vi "Remove Extra Blines.vi"(6 "Data In":u16[][](array[numeric]), 8 "#Aline":i32=400, 9 "Start index":i32, 10 "nAT per B":i32) -> (5 "Data Out":u16[][](array[numeric]))   [LabVIEW 2017]
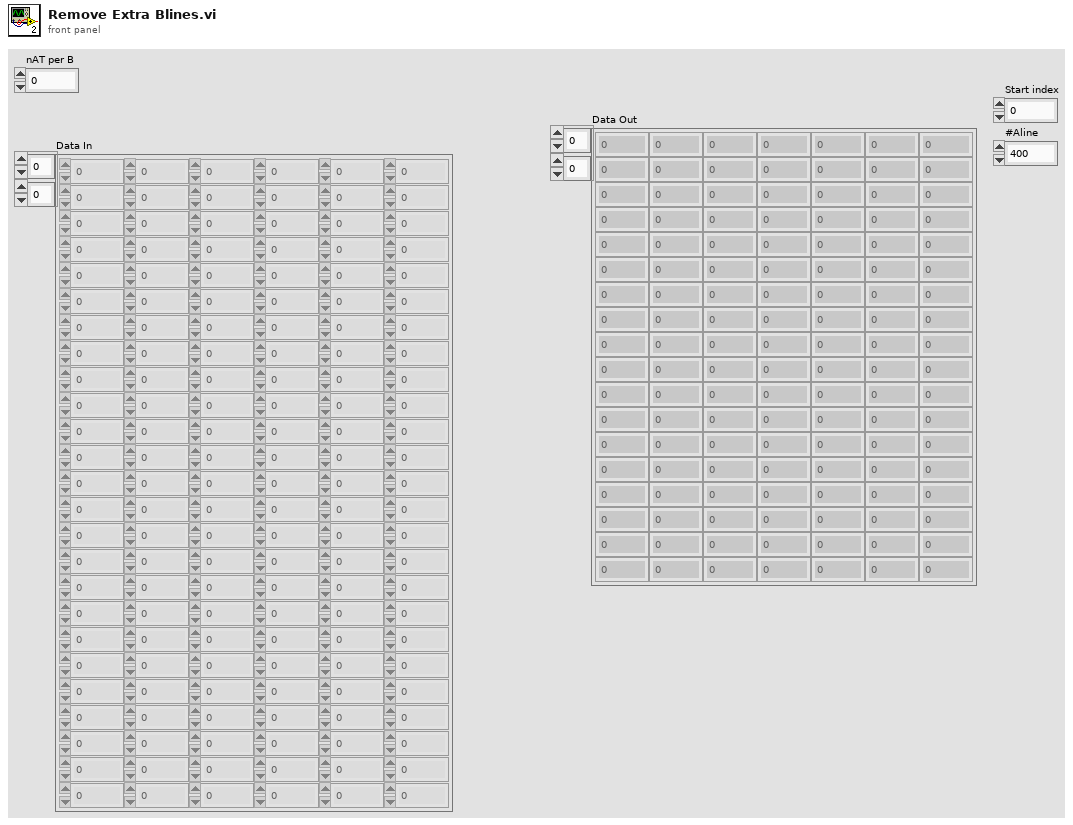
[diagram p1: front panel]
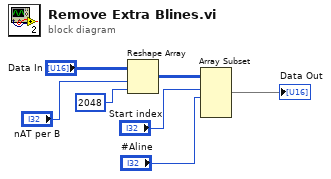
[diagram p0: block diagram]
diagram:
  n1 = Reshape Array("Data In", "nAT per B", 2048 ("dimension size")) -> (w5:u16[][])
  n2 = Array Subset(array=w5, index (row)="Start index", length (row)="#Aline") -> (→"Data Out":u16[][])  [unwired: 2 in]
